vi "Test.vi"() -> ()   [LabVIEW 2021]
panel:
  out "Array 4":i64[](array[numeric])=[1, 1, 8, 1, 5, 6, 7, 1, 1, 1, 7, 1, 2, 1]
  out "Max":i64[](array[numeric])=[9, 3, 9, 5, 9, 9, 9, 3, 4, 2, 9, 8, 9, 9]
  out "Array 2":i64[](array[numeric])=[21, 19, 17, 13, 12, 19, 15, 22, 17, 10, 16, 15, 18, 18]
  out "Array":cluster{"A":i64, "B":i64, "C":i64}[](array[cluster])=[{"A"=1, "B"=12, "C"=10}, {"A"=1, "B"=10, "C"=10}, {"A"=1, "B"=8, "C"=12}, {"A"=1, "B"=4, "C"=11}, {"A"=26, "B"=3, "C"=0}, {"A"=1, "B"=10, "C"=15}, {"A"=1, "B"=6, "C"=13}, {"A"=26, "B"=13, "C"=-12}, {"A"=26, "B"=8, "C"=-15}, {"A"=26, "B"=1, "C"=-15}, {"A"=26, "B"=7, "C"=-4}, {"A"=1, "B"=6, "C"=10}, {"A"=26, "B"=9, "C"=-5}, {"A"=26, "B"=9, "C"=-12}]
  in  "Input":string="inp w\nmul x 0\nadd x z\nmod x 26\ndiv z 1\nadd x 10\neql x w\neql x 0\nmul y 0\nadd y 25\nmul y x\nadd y 1\nmul z y\nmul y 0\nadd y w\nadd y 12\nmul y x\nadd z y\ninp w\nmul x 0\nadd x z\nmod x 26\ndiv z 1\nadd x 10\neql x w\neql x 0\nmul y 0\nadd y 25\nmul y x\nadd y 1\nmul z y\nmul y 0\nadd y w\nadd y 10\nmul y x\nadd z y\ninp w\nmul x 0\nadd x z\nmod x 26\ndiv z 1\nadd x 12\neql x w\neql x 0\nmul y 0\nadd y 25\nmul y x\nadd y 1\nmul z y\nmul y 0\nadd y w\nadd y 8\nmul y x\nadd z y\ninp w\nmul x 0\nadd x z\nmod x 26\ndiv z 1\nadd x 11\neql x w\neql x 0\nmul y 0\nadd y 25\nmul y x\nadd y 1\nmul z y\nmul y 0\nadd y w\nadd y 4\nmul y x\nadd z y\ninp w\nmul x 0\nadd x z\nmod x 26\ndiv z 26\nadd x 0\neql x w\neql x 0\nmul y 0\nadd y 25\nmul y x\nadd y 1\nmul z y\nmul y 0\nadd y w\nadd y 3\nmul y x\nadd z y\ninp w\nmul x 0\nadd x z\nmod x 26\ndiv z 1\nadd x 15\neql x w\neql x 0\nmul y 0\nadd y 25\nmul y x\nadd y 1\nmul z y\nmul y 0\nadd y w\nadd y 10\nmul y x\nadd z y\ninp w\nmul x 0\nadd x z\nmod x 26\ndiv z 1\nadd x 13\neql x w\neql x 0\nmul y 0\nadd y 25\nmul y x\nadd y 1\nmul z y\nmul y 0\nadd y w\nadd y 6\nmul y x\nadd z y\ninp w\nmul x 0\nadd x z\nmod x 26\ndiv z 26\nadd x -12\neql x w\neql x 0\nmul y 0\nadd y 25\nmul y x\nadd y 1\nmul z y\nmul y 0\nadd y w\nadd y 13\nmul y x\nadd z y\ninp w\nmul x 0\nadd x z\nmod x 26\ndiv z 26\nadd x -15\neql x w\neql x 0\nmul y 0\nadd y 25\nmul y x\nadd y 1\nmul z y\nmul y 0\nadd y w\nadd y 8\nmul y x\nadd z y\ninp w\nmul x 0\nadd x z\nmod x 26\ndiv z 26\nadd x -15\neql x w\neql x 0\nmul y 0\nadd y 25\nmul y x\nadd y 1\nmul z y\nmul y 0\nadd y w\nadd y 1\nmul y x\nadd z y\ninp w\nmul x 0\nadd x z\nmod x 26\ndiv z 26\nadd x -4\neql x w\neql x 0\nmul y 0\nadd y 25\nmul y x\nadd y 1\nmul z y\nmul y 0\nadd y w\nadd y 7\nmul y x\nadd z y\ninp w\nmul x 0\nadd x z\nmod x 26\ndiv z 1\nadd x 10\neql x w\neql x 0\nmul y 0\nadd y 25\nmul y x\nadd y 1\nmul z y\nmul y 0\nadd y w\nadd y 6\nmul y x\nadd z y\ninp w\nmul x 0\nadd x z\nmod x 26\ndiv z 26\nadd x -5\neql x w\neql x 0\nmul y 0\nadd y 25\nmul y x\nadd y 1\nmul z y\nmul y 0\nadd y w\nadd y 9\nmul y x\nadd z y\ninp w\nmul x 0\nadd x z\nmod x 26\ndiv z 26\nadd x -12\neql x w\neql x 0\nmul y 0\nadd y 25\nmul y x\nadd y 1\nmul z y\nmul y 0\nadd y w\nadd y 9\nmul y x\nadd z y"
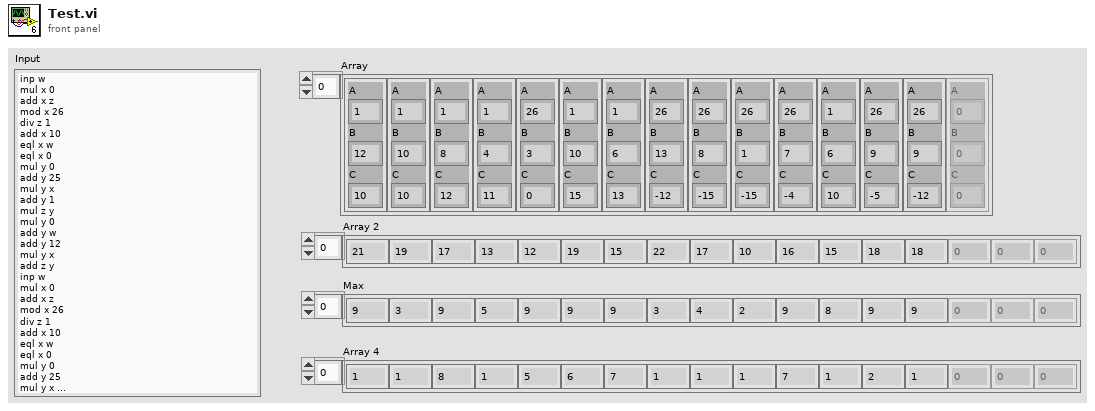
[diagram p1: front panel]
types:
  T1 = cluster{"default value 1":i64, "default value 1":i64, "default value 1":i64}
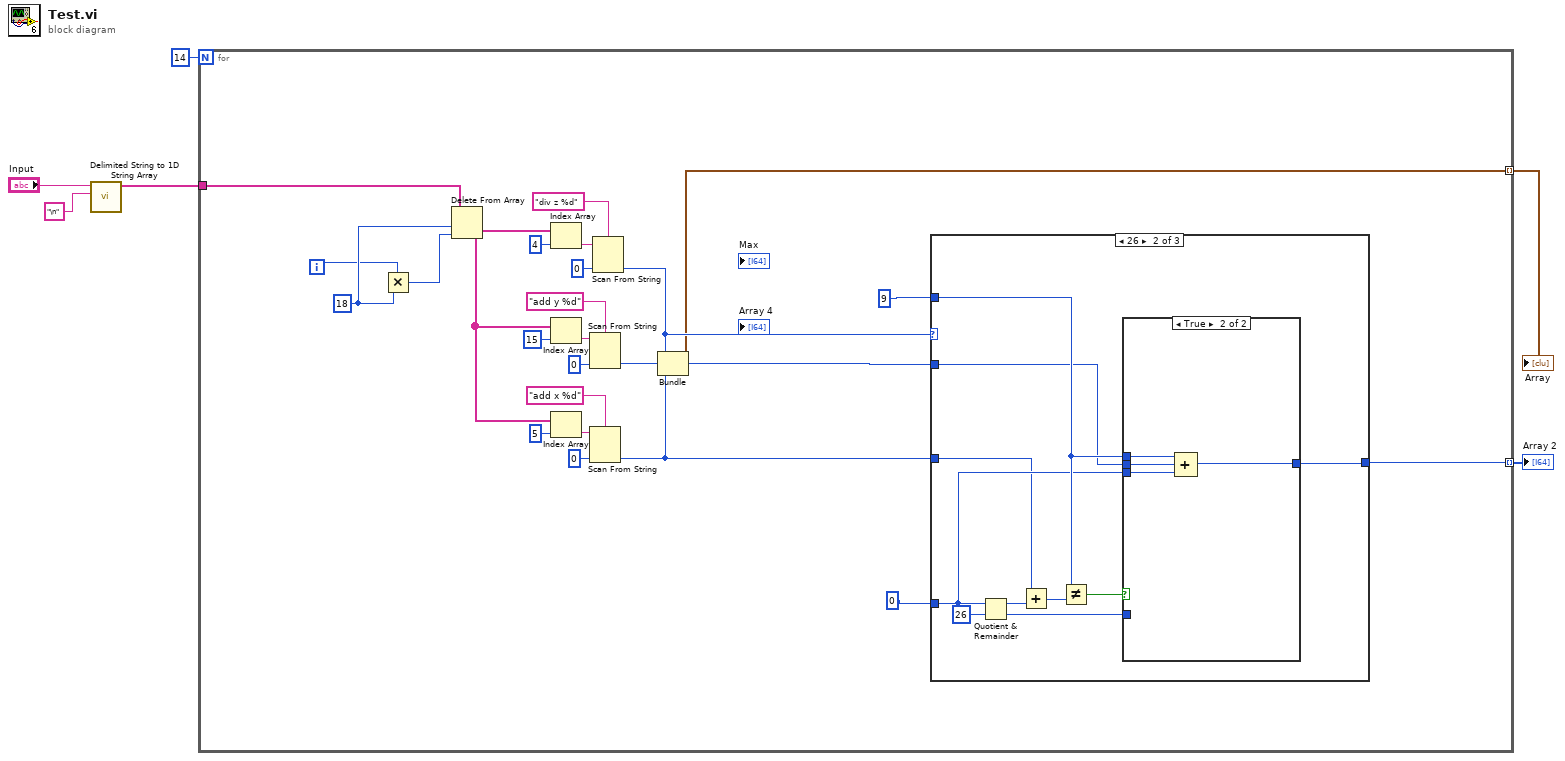
[diagram p0: block diagram]
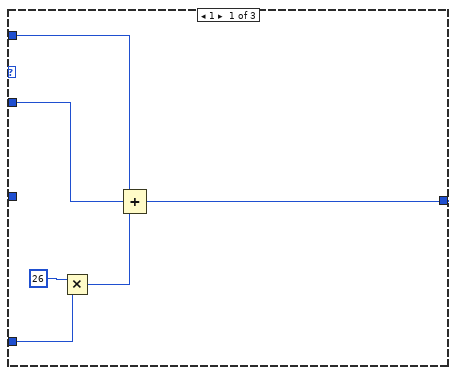
[diagram p2: hidden frame]
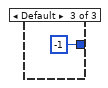
[diagram p4: hidden frame]
diagram:
  n1 = call <vilib>:"Delimited String to 1D String Array.vi"("delimiter"="\n", "delimited string"="Input") -> ("string array"=w4:string[])  [unwired: 9 in]
  n2 = for {
    N: 14 -> [_]
    tunnel: w4 -> [w18]
    tunnel: [w8] -> w1 mode=indexing
    tunnel: [w7] -> w2 mode=indexing
    i -> [w17]
    w20 = 18 ("length")
    n3 = Multiply(x=w17, y=w20) -> (x*y=w19:i32)
    n4 = Delete From Array(array=w18, length=w20, index=w19) -> (deleted portion=w21:string[])  [unwired: 1 out]
    n5 = Index Array(array=w21, index=4) -> (element=w16:string)
    n6 = Index Array(array=w21, index=15) -> (element=w28:string)
    n7 = Index Array(array=w21, index=5) -> (element=w23:string)
    n8 = Scan From String(format string="add y %d" ("y"), input string=w28, default 1=i64 0 ("default value 1")) -> (output 1=w10:i64)  [unwired: 2 in, 3 out]
    n9 = Scan From String(format string="add x %d" ("y"), input string=w23, default 1=i64 0 ("default value 1")) -> (output 1=w9:i64)  [unwired: 2 in, 3 out]
    n10 = Scan From String(format string="div z %d" ("y"), input string=w16, default 1=i64 0 ("default value 1")) -> (output 1=w12:i64)  [unwired: 2 in, 3 out]
    n11 = Bundle("default value 1"=w12, "default value 1"=w10, "default value 1"=w9) -> (w7:T1)  [unwired: 1 in]
    n12 = case shown="26" w12 {
      tunnel: 9 -> [w34 w42 _]
      tunnel: 0 -> [w36 w39 _]
      tunnel: [w32 w41 i64 -1] -> w8
      tunnel: w10 -> [w31 w37 _]
      tunnel: w9 -> [_ w38 _]
      frame 1 {
        n13 = Multiply(x=i64 26 ("y"), y=w36) -> (x*y=w33:i64)
        n14 = Compound Arithmetic op=ADD(w34, w31, w33) -> (w32:i64)
      }
      frame 26 {
        n15 = Quotient & Remainder(x=w39, y=i64 26) -> (x-y*floor(x/y)=w45:i64, floor(x/y)=w40:i64)
        n16 = Add(x=w38, y=w45) -> (x+y=w44:i64)
        n17 = Not Equal?(x=w42, y=w44) -> (x != y?=w43:bool)
        n18 = case shown="True" w43 {
          tunnel: w42 -> [_ w51]
          tunnel: [w47 w50] -> w41
          tunnel: w40 -> [w47 _]
          tunnel: w39 -> [_ w49]
          tunnel: w37 -> [_ w48]
          frame False {
          }
          frame True {
            n19 = Compound Arithmetic op=ADD(w51, w48, w49) -> (w50:i64)
          }
        }
      }
      frame Default {
      }
    }
  }
  "Array" <- w2
  "Array 2" <- w1
